vi "Panel Reset Gas Vol.vi"(11 "Tasks In":refnum<k21>[](array[refnum])) -> (3 "CDAQ Data Out":dbl[](array[numeric]))   [LabVIEW 2012]
panel:
  in  "ok":bool
  out "message":string="Reset Gas Volume"
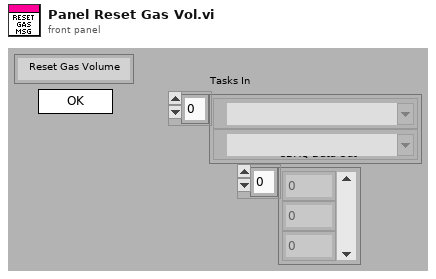
[diagram p1: front panel]
types:
  T1 = enum16{"Exe", "Init CDAQ", "Gather DATA", "Close"}
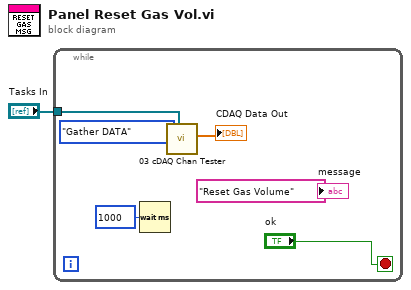
[diagram p0: block diagram]
diagram:
  n1 = while {
    tunnel: "Tasks In" -> [w4]
    stop <- "ok" stop-if-true
    n2 = Wait (ms)(milliseconds to wait=u32 1000) -> ()  [unwired: 1 out]
    n3 = call "03 cDAQ Chan Tester.vi"("Tasks In"=w4, "Mode"=T1."Gather DATA") -> ("CDAQ Data Out"=→"CDAQ Data Out":dbl[])  [unwired: 7 in, 2 out]
    "message" <- "Reset Gas Volume" ("message")
  }
